vi "SimulatedConfigureSweep.vi"(8 "error in (no error)":errorcluster, 10 "channels in data group":T1[](array[typedef]), 11 "AssetNodes":T4[](array[typedef])) -> (0 "error out":errorcluster)   [LabVIEW 2017, in "EmsaAcquisition.lvlib"]
uses:
  <vilib>/addons/InsightCM/Devices/Shared/Emsa/EmsaAcquisition/EmsaAcquisition.lvlib
  <vilib>/addons/InsightCM/MessageBus/Base/controls/AssetNode.ctl
  <vilib>/addons/InsightCM/MessageBus/Base/controls/AssetState.ctl
  <vilib>/addons/InsightCM/MessageBus/Base/controls/KeyValuePair.ctl
  <vilib>/addons/InsightCM/MessageBus/Base/controls/OperatingState.ctl
  <vilib>/addons/InsightCM/MessageBus/Base/controls/Trigger.ctl
  <vilib>/addons/InsightCM/MessageBus/Base/controls/Condition.ctl
  <vilib>/addons/InsightCM/MessageBus/Base/controls/Metric.ctl
  <vilib>/addons/InsightCM/MessageBus/Base/controls/TrendAlarmRule.ctl
  <vilib>/addons/InsightCM/MessageBus/Base/controls/TrendAlarmLevel.ctl
  <vilib>/addons/InsightCM/MessageBus/Base/controls/AlarmAction.ctl
  <vilib>/addons/InsightCM/MessageBus/Base/controls/AssetNodeReference.ctl
  <vilib>/addons/InsightCM/MessageBus/Base/controls/R2_Channel.ctl
  <vilib>/addons/InsightCM/Devices/Shared/Emsa/EmsaAcquisition/controls/SweepElement.ctl
  <vilib>/addons/InsightCM/Devices/Shared/Emsa/EmsaAcquisition/controls/SimulatedSweepConfig.ctl
  <vilib>/addons/InsightCM/Devices/Shared/Emsa/EmsaAcquisition/subVIs/SimulatedConfigRefGlobal.vi
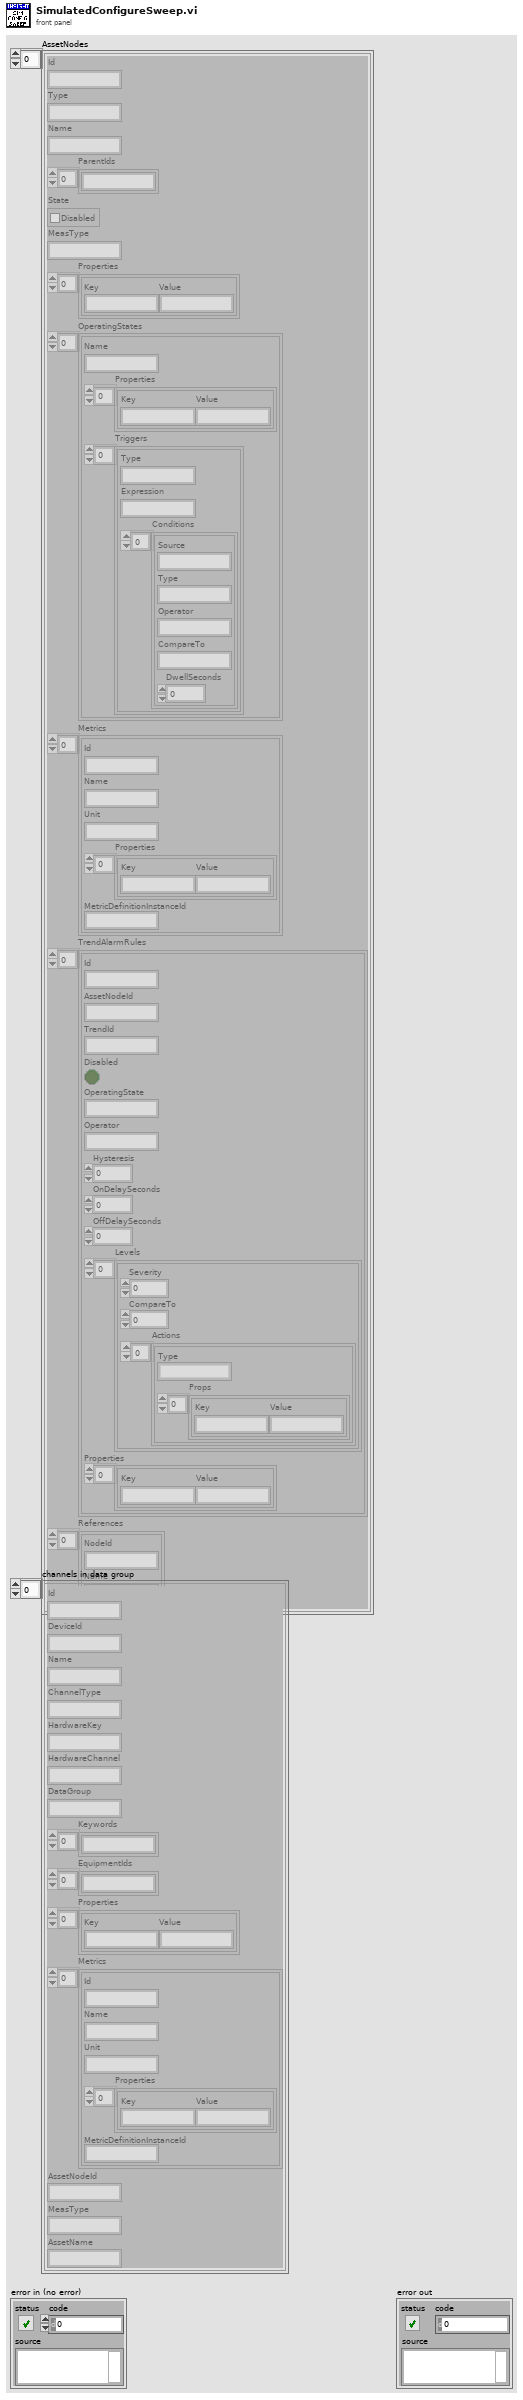
[diagram p1: front panel]
types:
  T1 = typedef "R2_Channel.ctl" = cluster{"Id":string, "DeviceId":string, "Name":string, "ChannelType":string, "HardwareKey":string, "HardwareChannel":string, "DataGroup":string, "Keywords":string[], "EquipmentIds":string[], "Properties":T2[], "Metrics":T3[], "AssetNodeId":string, "MeasType":string, "AssetName":string}
  T2 = typedef "KeyValuePair.ctl" = cluster{"Key":string, "Value":string}
  T3 = typedef "Metric.ctl" = cluster{"Id":string, "Name":string, "Unit":string, "Properties":T2[], "MetricDefinitionInstanceId":string}
  T4 = typedef "AssetNode.ctl" = cluster{"Id":string, "Type":string, "Name":string, "ParentIds":string[], "State":T5, "MeasType":string, "Properties":T2[], "OperatingStates":T6[], "Metrics":T3[], "TrendAlarmRules":T9[], "References":T12[]}
  T5 = typedef "AssetState.ctl" = cluster{"Disabled":bool}
  T6 = typedef "OperatingState.ctl" = cluster{"Name":string, "Properties":T2[], "Triggers":T7[]}
  T7 = typedef "Trigger.ctl" = cluster{"Type":string, "Expression":string, "Conditions":T8[]}
  T8 = typedef "Condition.ctl" = cluster{"Source":string, "Type":string, "Operator":string, "CompareTo":string, "DwellSeconds":dbl}
  T9 = typedef "TrendAlarmRule.ctl" = cluster{"Id":string, "AssetNodeId":string, "TrendId":string, "Disabled":bool, "OperatingState":string, "Operator":string, "Hysteresis":dbl, "OnDelaySeconds":dbl, "OffDelaySeconds":dbl, "Levels":T10[], "Properties":T2[]}
  T10 = typedef "TrendAlarmLevel.ctl" = cluster{"Severity":i32, "CompareTo":dbl, "Actions":T11[]}
  T11 = typedef "AlarmAction.ctl" = cluster{"Type":string, "Props":T2[]}
  T12 = typedef "AssetNodeReference.ctl" = cluster{"NodeId":string, "Name":string}
  T13 = typedef "EmsaAcquisition.lvlib/SweepElement.ctl" = cluster{"Frequency":dbl, "Amplitude":dbl}
  T14 = typedef "EmsaAcquisition.lvlib/SimulatedConfigRefs.ctl" = cluster{"SimulatedSignalConfig":refnum<vi>}
  T15 = typedef "EmsaAcquisition.lvlib/SimulatedSignalConfig.ctl" = cluster{"Channel Name":string[], "Valid":bool[], "Hardware Channel":string[], "Unit":string[], "Sweep Configs":T16[]}
  T16 = typedef "EmsaAcquisition.lvlib/SimulatedSweepConfig.ctl" = cluster{"Sweep Frequency List":cluster{"frequency":dbl, "bandwidth":dbl}[], "Detection Time":dbl, "Detection Mode":enum16{"Peak", "Quasi Peak", "Average"}, "Full Scale Volts":dbl, "Total Sweep Pts":i32, "Sweep Pointer":i32, "Sweep":T13[], "Sweep Start Time":timestamp}
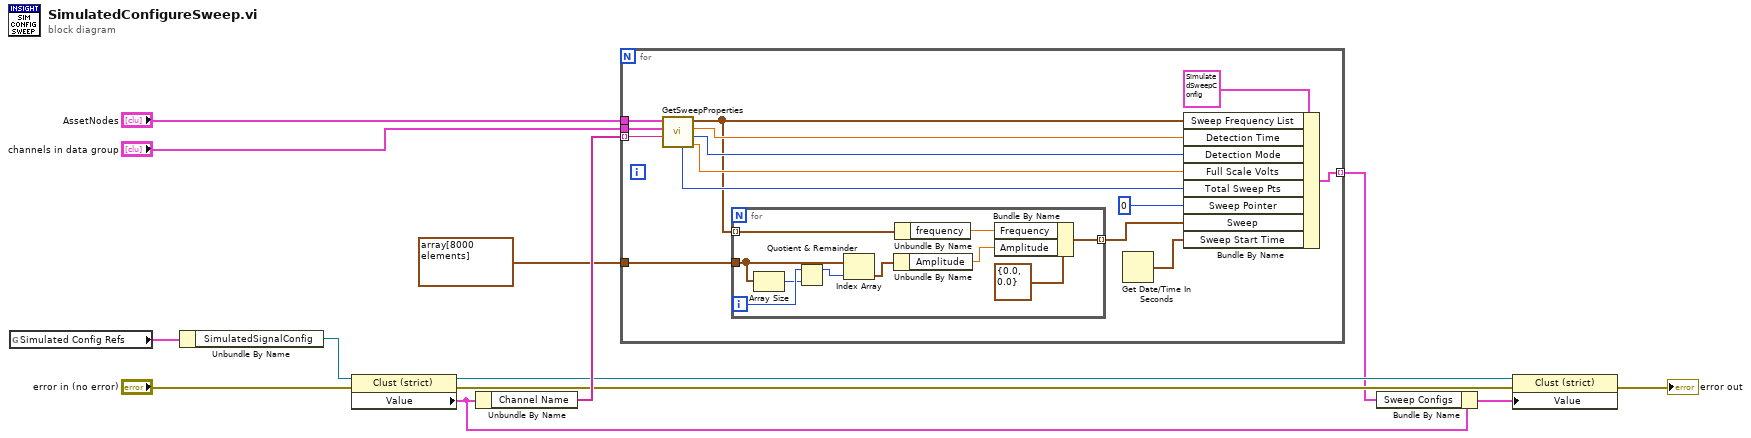
[diagram p0: block diagram]
diagram:
  n1 = global read "SimulatedConfigRefGlobal.vi" "Simulated Config Refs"() -> (w11:T14)
  n2 = Unbundle By Name(w11) -> ("SimulatedSignalConfig"=w9:refnum<vi>)
  n3 = property class="Clust (strict)"(reference=w9, error in="error in (no error)") -> (reference out=w6:refnum<vi>, error out=w4:errorcluster, "Value"=w7:T15)
  n4 = Unbundle By Name(w7) -> ("Channel Name"=w8:string[])
  n5 = for {
    tunnel: "AssetNodes" -> [w27]
    tunnel: "channels in data group" -> [w26]
    tunnel: w8 -> [w25] mode=indexing
    tunnel: [w20] -> w2 mode=indexing
    tunnel: T13[] array[8000 elements] -> [w14]
    n6 = call <vilib>:"GetSweepProperties.vi"("channel"=w25, "data group channels"=w26, "asset nodes"=w27) -> ("full scale voltage"=w21:dbl, "DetectionMode"=w22:enum16{"Peak", "Quasi Peak", "Average"}, "detection time"=w23:dbl, "sweep freq list"=w17:cluster{"frequency":dbl, "bandwidth":dbl}[], "total number of sweep points"=w18:i32)  [unwired: 4 in]
    n7 = for {
      tunnel: w17 -> [w37] mode=indexing
      tunnel: [w34] -> w16 mode=indexing
      tunnel: w14 -> [w32]
      i -> [w29]
      n8 = Array Size(array=w32) -> (size(s)=w28:i32)
      n9 = Quotient & Remainder(x=w29, y=w28) -> (x-y*floor(x/y)=w31:i32)  [unwired: 1 out]
      n10 = Index Array(array=w32, index=w31) -> (element=w30:T13)
      n11 = Unbundle By Name(w30) -> ("Amplitude"=w33:dbl)
      n12 = Unbundle By Name(w37) -> ("frequency"=w35:dbl)
      n13 = Bundle By Name(cluster=T13 {"Frequency"=0.0, "Amplitude"=0.0} ("Current Point"), "Frequency"=w35, "Amplitude"=w33) -> (w34:T13)
    }
    n14 = Get Date/Time In Seconds() -> (seconds since 1Jan1904=w15:timestamp)
    n15 = Bundle By Name(cluster=T16 {"Sweep Frequency List"=[], "Detection Time"=0.0, "Detection Mode"=enum."Peak", "Full Scale Volts"=0.0, "Total Sweep Pts"=0, "Sweep Pointer"=0, "Sweep"=[], "Sweep Start Time"=timestamp(0 s since 1904-01-01)} ("Cluster"), "Sweep Frequency List"=w17, "Detection Time"=w23, "Detection Mode"=w22, "Full Scale Volts"=w21, "Total Sweep Pts"=w18, "Sweep Pointer"=0, "Sweep"=w16, "Sweep Start Time"=w15) -> (w20:T16)
  }
  n16 = Bundle By Name(cluster=w7, "Sweep Configs"=w2) -> (w5:T15)
  n17 = property class="Clust (strict)"(reference=w6, error in=w4, "Value"=w5) -> (error out=→"error out":errorcluster)  [unwired: 1 out]
